vi "resetCurrentOutputState.vi"(8 "error in (no error)":errorcluster, 11 "AnalogOutput in":refnum<class "AnalogOutput.lvclass">) -> (0 "error out":errorcluster, 3 "AnalogOutput out":refnum<class "AnalogOutput.lvclass">)   [LabVIEW 2011, in "Hardware.lvlib" / "Channels.lvlib" / "AnalogOutput.lvclass"]
uses:
  AnalogOutput.lvclass
  AnalogOutput.lvclass/AnalogOutput.ctl
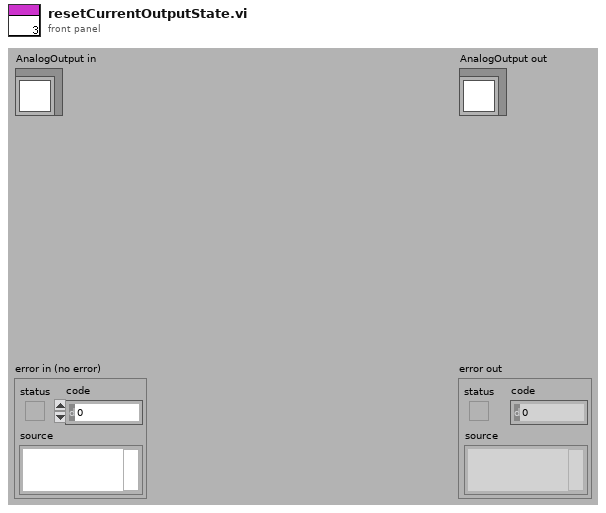
[diagram p1: front panel]
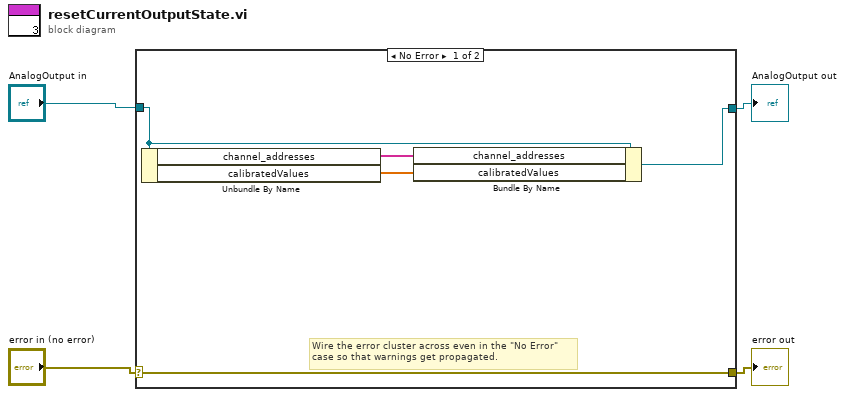
[diagram p0: block diagram]
diagram:
  n1 = case shown="No Error" "error in (no error)" {
    selector: "error in (no error)" -> [w9 w11]
    tunnel: [w9 w11] -> w2
    tunnel: [w6 w10] -> w3
    tunnel: "AnalogOutput in" -> [w5 w10]
    frame No Error {
      # "Wire the error cluster across even in the \"No Error\"\ncase so that warnings get propagated."
      n2 = Unbundle By Name(w5) -> ("channel_addresses"=w8:string[], "calibratedValues"=w7:dbl[])
      n3 = Bundle By Name(cluster=w5, "channel_addresses"=w8, "calibratedValues"=w7) -> (w6:refnum<class "AnalogOutput.lvclass">)
    }
    frame Error {
    }
  }
  "error out" <- w2
  "AnalogOutput out" <- w3
